vi "Set FIeld mercury.vi"(5 "wait for hold":bool, 6 "FIeld mT":dbl, 7 "FIeld mT  per sec":dbl, 8 "error in (no error)":errorcluster, 10 "Device on PSU":string, 11 "VISA resource name":refnum<visa-resource-name>) -> (0 "error out":errorcluster, 2 "Current FIeld mT":dbl, 3 "VISA resource name out":refnum<visa-resource-name>)   [LabVIEW 2024]
panel:
  out "Array":string[](array[string])
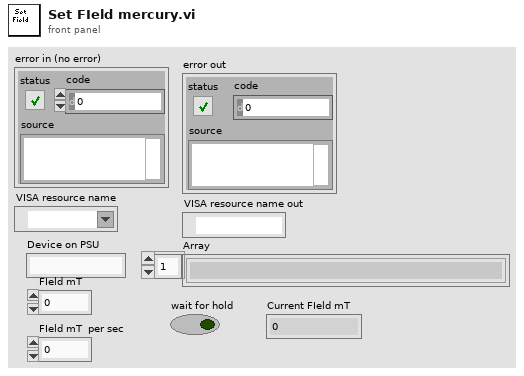
[diagram p1: front panel]
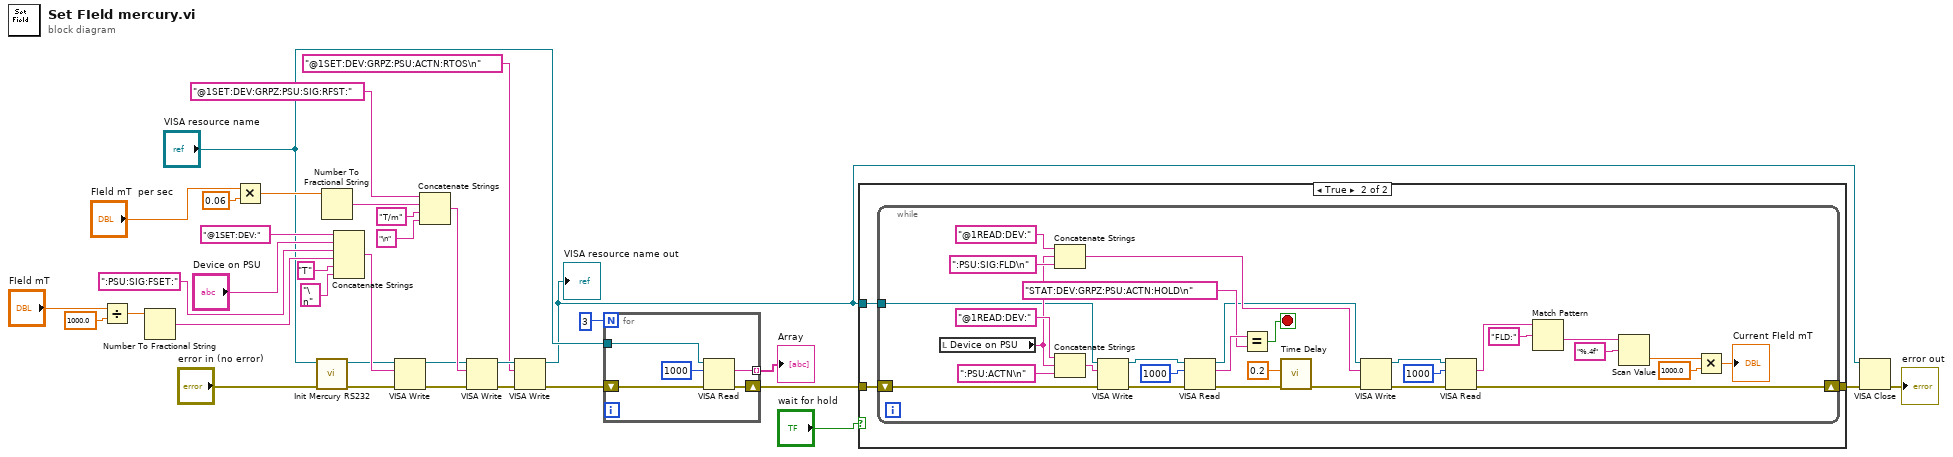
[diagram p0: block diagram]
diagram:
  n1 = Divide(x="FIeld mT", y=1000.0) -> (x/y=w28:dbl)
  n2 = Number To Fractional String(number=w28) -> (F-format string=w30:string)  [unwired: 3 in]
  n3 = Multiply(x="FIeld mT  per sec", y=0.06) -> (x*y=w21:dbl)
  n4 = call "Init Mercury RS232.vi"("error in (no error)"="error in (no error)", "VISA resource name"="VISA resource name") -> ("error out"=w13:errorcluster, "VISA resource name out"=w14:refnum<visa-resource-name>)  [unwired: 8 in]
  n5 = Number To Fractional String(number=w21) -> (F-format string=w20:string)  [unwired: 3 in]
  n6 = Concatenate Strings("@1SET:DEV:" ("string"), "Device on PSU", ":PSU:SIG:FSET:" ("string"), w30, "T" ("string"), "\n" ("string")) -> (w32:string)
  n7 = VISA Write(VISA resource name=w14, write buffer=w32, error in (no error)=w13) -> (VISA resource name out=w12:refnum<visa-resource-name>, error out=w10:errorcluster)  [unwired: 1 out]
  n8 = Concatenate Strings("@1SET:DEV:GRPZ:PSU:SIG:RFST:" ("string"), w20, "T/m" ("string"), "\n" ("string")) -> (w29:string)
  n9 = VISA Write(VISA resource name=w12, write buffer=w29, error in (no error)=w10) -> (VISA resource name out=w17:refnum<visa-resource-name>, error out=w7:errorcluster)  [unwired: 1 out]
  n10 = VISA Write(VISA resource name=w17, write buffer="@1SET:DEV:GRPZ:PSU:ACTN:RTOS\n", error in (no error)=w7) -> (VISA resource name out=w2:refnum<visa-resource-name>, error out=w6:errorcluster)  [unwired: 1 out]
  "VISA resource name out" <- w2
  n11 = for {
    N: 3 -> [_]
    tunnel: "VISA resource name" -> [w40]
    tunnel: [w36] -> w9 mode=indexing
    shift-right: [w37] -> w5
    shift-left: w6 -> [w38]
    n12 = VISA Read(VISA resource name=w40, byte count=u32 1000, error in (no error)=w38) -> (read buffer=w36:string, error out=w37:errorcluster)  [unwired: 2 out]
  }
  "Array" <- w9
  n13 = case shown="True" "wait for hold" {
    tunnel: w5 -> [w41 w44]
    tunnel: [w41 w43] -> w3
    tunnel: w2 -> [_ w42]
    frame False {
    }
    frame True {
      n14 = while {
        shift-right: [w47] -> w43
        shift-left: w44 -> [w64]
        tunnel: w42 -> [w46]
        stop <- w63 stop-if-true
        n15 = local read "Device on PSU"() -> (w48:string)
        n16 = Concatenate Strings("@1READ:DEV:" ("string"), w48, ":PSU:SIG:FLD\n" ("string")) -> (w56:string)
        n17 = Concatenate Strings("@1READ:DEV:" ("write buffer"), w48, ":PSU:ACTN\n" ("string")) -> (w72:string)
        n18 = VISA Write(VISA resource name=w46, write buffer=w72, error in (no error)=w64) -> (VISA resource name out=w69:refnum<visa-resource-name>, error out=w71:errorcluster)  [unwired: 1 out]
        n19 = VISA Read(VISA resource name=w69, byte count=u32 1000, error in (no error)=w71) -> (VISA resource name out=w45:refnum<visa-resource-name>, read buffer=w67:string, error out=w70:errorcluster)  [unwired: 1 out]
        n20 = Equal?(x=w67, y="STAT:DEV:GRPZ:PSU:ACTN:HOLD\n") -> (x = y?=w63:bool)
        n21 = call "Time Delay"("error in (no error)"=w70, "Delay Time (s)"=0.2) -> ("error out"=w49:errorcluster)  [unwired: 9 in]
        n22 = VISA Write(VISA resource name=w45, write buffer=w56, error in (no error)=w49) -> (VISA resource name out=w57:refnum<visa-resource-name>, error out=w58:errorcluster)  [unwired: 1 out]
        n23 = VISA Read(VISA resource name=w57, byte count=u32 1000, error in (no error)=w58) -> (read buffer=w61:string, error out=w47:errorcluster)  [unwired: 2 out]
        n24 = Match Pattern(string=w61, regular expression="FLD:") -> (after substring=w62:string)  [unwired: 1 in, 3 out]
        n25 = Scan Value(string=w62, format string="%.4f") -> (value=w59:dbl)  [unwired: 1 in, 1 out]
        n26 = Multiply(x=w59, y=1000.0) -> (x*y=→"Current FIeld mT":dbl)
      }
    }
  }
  n27 = VISA Close(VISA resource name=w2, error in (no error)=w3) -> (error out=→"error out":errorcluster)
